vi "LabVIEW DataType to Measurement DataType.vi"(1 "LabVIEW type":T2) -> (0 "Measurement DataType":T1)   [LabVIEW 2020, in "Measurement Client Wrapper.lvclass"]
uses:
  Measurement Client Wrapper.lvclass
  <vilib>/Utility/Data Type/Type Definitions/Data Type.ctl
  <vilib>/TAF/LabVIEW Measurement Client/RPC Messages/ni_measurements_v1_Type.ctl
  <vilib>/Utility/Data Type/NI_Data Type.lvlib
  <vilib>/TAF/LabVIEW Measurement Client/Measurement_client-release.lvlib
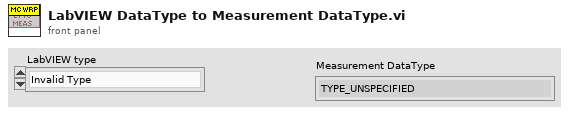
[diagram p1: front panel]
types:
  T1 = typedef "Measurement_client-release.lvlib/ni_measurements_v1_Type.ctl" = enum32{"TYPE_UNSPECIFIED", "TYPE_DOUBLE", "TYPE_FLOAT", "TYPE_INT64", "TYPE_UINT64", "TYPE_INT32", "TYPE_FIXED64", "TYPE_FIXED32", "TYPE_BOOL", "TYPE_STRING", "TYPE_GROUP", "TYPE_MESSAGE", "TYPE_BYTES", "TYPE_UINT32", "TYPE_ENUM", "TYPE_SFIXED32", "TYPE_SFIXED64", "TYPE_SINT32", "TYPE_SINT64"}
  T2 = typedef "NI_Data Type.lvlib/Data Type.ctl" = enum8{"Invalid Type", "Void", "I8", "I16", "I32", "I64", "U8", "U16", "U32", "U64", "Single Float", "Double Float", "Extended Float", "Single Complex", "Double Complex", "Extended Complex", "Enum U8", "Enum U16", "Enum U32", "Enum U64", "Single Float With Unit", "Double Float With Unit", "Extended Float With Unit", "Single Complex with Unit", "Double Complex with Unit", "Extended Complex with Unit", "Boolean", "String", "Path", "Picture", "Tag", "Array", "Cluster", "Variant", "LV Variant", "Waveform", "Timestamp", "Digital Waveform", "Digital Data", "ExpressData", "Refnum", "External Data", "VI", "Poly VI", "LabVIEW Class Instance", "Fixed Point", "Set Collection", "Map Collection"}
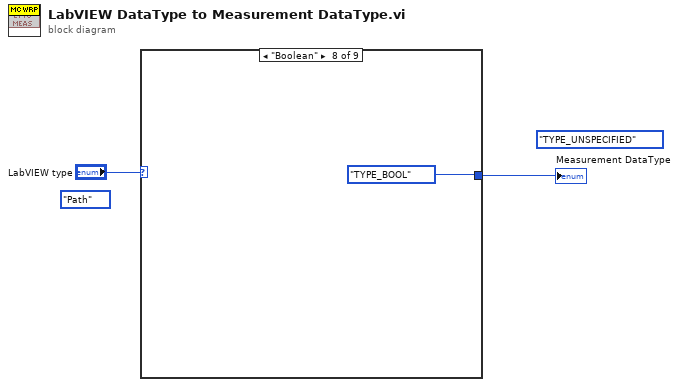
[diagram p0: block diagram]
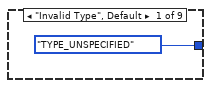
[diagram p2: hidden frame]
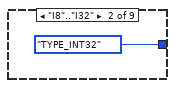
[diagram p3: hidden frame]
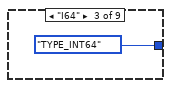
[diagram p4: hidden frame]
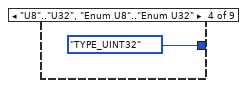
[diagram p5: hidden frame]
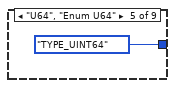
[diagram p6: hidden frame]
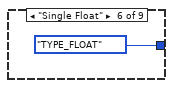
[diagram p7: hidden frame]
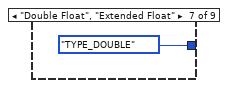
[diagram p8: hidden frame]
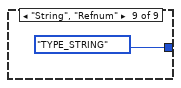
[diagram p9: hidden frame]
diagram:
  (unwired) ni_measurements_v1_Type."TYPE_UNSPECIFIED" ("Measurement DataType")
  (unwired) Data_Type."Path" ("LabVIEW type")
  n1 = case shown="\"Boolean\"" "LabVIEW type" {
    tunnel: [ni_measurements_v1_Type."TYPE_UNSPECIFIED" ("Measurement DataType") ni_measurements_v1_Type."TYPE_INT32" ("Measurement DataType") ni_measurements_v1_Type."TYPE_INT64" ("Measurement DataType") ni_measurements_v1_Type."TYPE_UINT32" ("Measurement DataType") ni_measurements_v1_Type."TYPE_UINT64" ("Measurement DataType") ni_measurements_v1_Type."TYPE_FLOAT" ("Measurement DataType") ni_measurements_v1_Type."TYPE_DOUBLE" ("Measurement DataType") ni_measurements_v1_Type."TYPE_BOOL" ("Measurement DataType") ni_measurements_v1_Type."TYPE_STRING" ("Measurement DataType")] -> w1
    frame "Invalid Type", Default {
    }
    frame "I8".."I32" {
    }
    frame "I64" {
    }
    frame "U8".."U32", "Enum U8".."Enum U32" {
    }
    frame "U64", "Enum U64" {
    }
    frame "Single Float" {
    }
    frame "Double Float", "Extended Float" {
    }
    frame "Boolean" {
    }
    frame "String", "Refnum" {
    }
  }
  "Measurement DataType" <- w1
